vi "Auto 5.vi"(8 "Error In":errorcluster) -> (0 "Error Out":errorcluster)   [LabVIEW 2014]
uses:
  Robot Global Data.vi
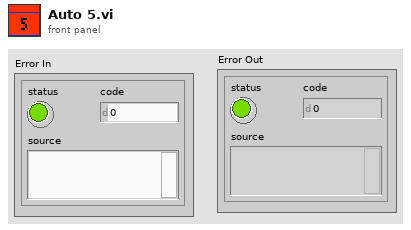
[diagram p1: front panel]
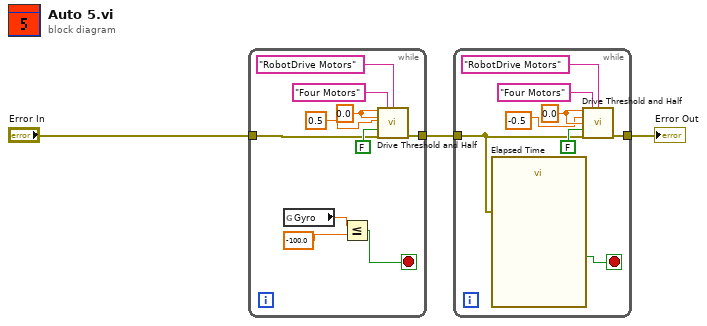
[diagram p0: block diagram]
diagram:
  n1 = while {
    tunnel: "Error In" -> [w10]
    tunnel: [w9] -> w3
    stop <- w4 stop-if-true
    w8 = 0.0 ("Arm Value")
    n2 = global read "Robot Global Data.vi" "Gyro"() -> (w6:dbl)
    n3 = Less Or Equal?(x=w6, y=-100.0) -> (x <= y?=w4:bool)
    n4 = call "Drive Threshold and Half.vi"("X In"=w8, "Drive refnum name"="Four Motors" ("refnum name"), "Send to DB Name"="RobotDrive Motors" ("Name"), "Y In"=w8, "R In"=0.5 ("X In"), "Speed Toggle"=FALSE ("Grabber Open/Close"), "Error In"=w10) -> ("Error Out"=w9:errorcluster)  [unwired: 8 in]
  }
  n5 = while {
    tunnel: w3 -> [w14]
    tunnel: [w18] -> w2
    stop <- w15 stop-if-true
    w17 = 0.0 ("Arm Value")
    n6 = call "Elapsed Time"("error in (no error)"=w14) -> ("Time has Elapsed"=w15:bool)  [unwired: 11 in, 7 out]
    n7 = call "Drive Threshold and Half.vi"("X In"=w17, "Drive refnum name"="Four Motors" ("refnum name"), "Send to DB Name"="RobotDrive Motors" ("Name"), "Y In"=-0.5 ("X In"), "R In"=w17, "Speed Toggle"=FALSE ("Grabber Open/Close"), "Error In"=w14) -> ("Error Out"=w18:errorcluster)  [unwired: 8 in]
  }
  "Error Out" <- w2
